vi "Pulses.vi"(3 "error in (no error)":errorcluster, 4 "try connection?":bool, 5 "VISA resource name in":refnum<visa-resource-name>) -> (0 "error out":errorcluster, 1 "connection result":cluster{"pulses":i32, "connected":bool}, 2 "VISA resource name out":refnum<visa-resource-name>)   [LabVIEW 2011]
doc: "Connects to the given serial port, check if there is an appropriately programmed Arduino listening on it, and if so reports the number of pulses per revolution."
uses:
  <vilib>/Instr/_visa.llb/VISA Configure Serial Port (Instr).vi
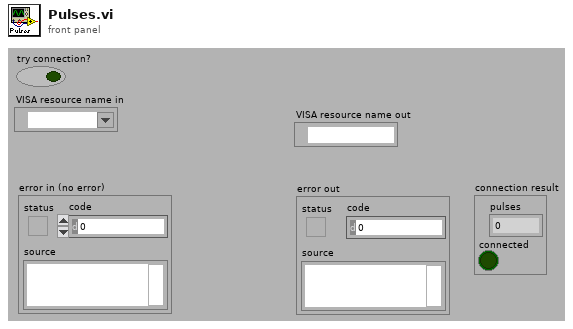
[diagram p1: front panel]
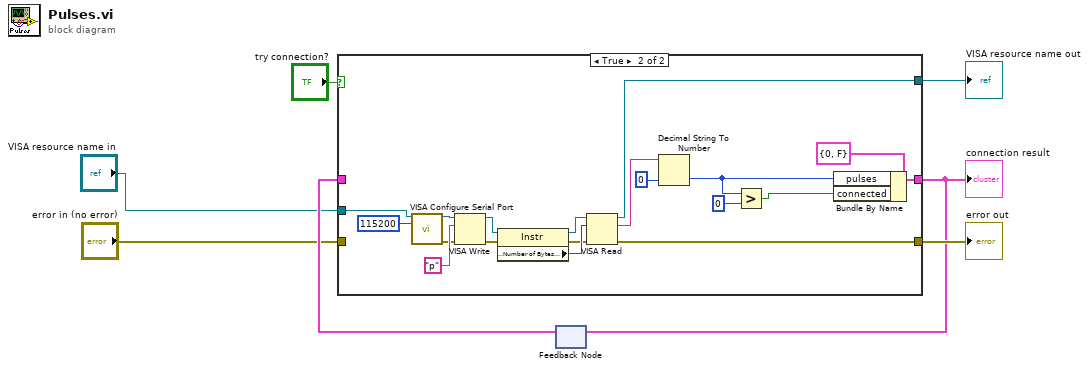
[diagram p0: block diagram]
diagram:
  n1 = feedback #1() -> (w4:cluster{"pulses":i32, "connected":bool})  [unwired: 1 in]
  n2 = case shown="True" "try connection?" {
    tunnel: [w8 w17] -> w5
    tunnel: [w10 w16] -> w7
    tunnel: [w9 w15] -> w6
    tunnel: w4 -> [w8 _]
    tunnel: "VISA resource name in" -> [w10 w14]
    tunnel: "error in (no error)" -> [w9 _]
    frame False {
    }
    frame True {
      n3 = call-poly "VISA Configure Serial Port"("VISA resource name"=w14, "baud rate (9600)"=u32 115200) -> ("VISA resource name out"=w21:refnum<visa-resource-name>, "error out"=w20:errorcluster)  [unwired: 12 in]
      n4 = VISA Write(VISA resource name=w21, write buffer="p", error in (no error)=w20) -> (VISA resource name out=w27:refnum<visa-resource-name>, error out=w28:errorcluster)  [unwired: 1 out]
      n5 = property class="Instr"(reference=w27, error in=w28) -> (reference out=w26:refnum<visa-resource-name>, error out=w24:errorcluster, "Serial Settings:Number of Bytes at Serial Port"=w25:u32)
      n6 = VISA Read(VISA resource name=w26, byte count=w25, error in (no error)=w24) -> (VISA resource name out=w16:refnum<visa-resource-name>, read buffer=w23:string, error out=w15:errorcluster)  [unwired: 1 out]
      n7 = Decimal String To Number(string=w23, default (0L)=u32 0 ("default (0 I32)")) -> (number=w13:u32)  [unwired: 1 in, 1 out]
      n8 = Greater?(x=w13, y=u32 0) -> (0:w11:bool)
      n9 = Bundle By Name(cluster=cluster{"pulses":i32, "connected":bool} {"pulses"=0, "connected"=FALSE} ("input cluster"), "pulses"=w13, "connected"=w11) -> (w17:cluster{"pulses":i32, "connected":bool})
    }
  }
  "error out" <- w6
  "VISA resource name out" <- w7
  "connection result" <- w5
  n10 = feedback-in #1(w5) -> ()
